vi "Format Coordinates.vi"(11 "1D String Array":string[](array[string])) -> (3 "Coordinates":i32[][](array[numeric]))   [LabVIEW 2019]
doc: "Given a 1D string array of points, turn them into a 2D array of coordinates."
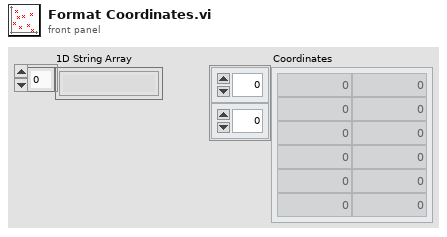
[diagram p1: front panel]
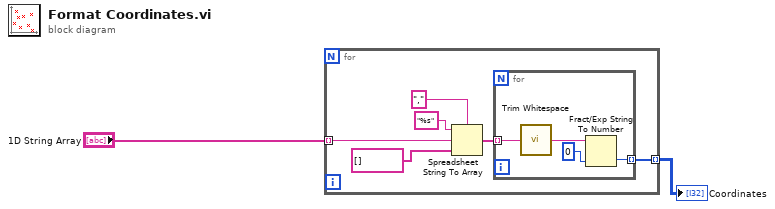
[diagram p0: block diagram]
diagram:
  n1 = for {
    tunnel: "1D String Array" -> [w8] mode=indexing
    tunnel: [w3] -> w2 mode=indexing
    n2 = Spreadsheet String To Array(delimiter (Tab)="," ("delimiter"), format string="%s", spreadsheet string=w8, array type (2D Dbl)=string[] []) -> (array=w5:string[])
    n3 = for {
      tunnel: w5 -> [w12] mode=indexing
      tunnel: [w9] -> w3 mode=indexing
      n4 = call <vilib>:"Trim Whitespace.vi"("string"=w12) -> ("trimmed string"=w11:string)  [unwired: 1 in]
      n5 = Fract/Exp String To Number(string=w11, default (0 dbl)=0 ("default (0 DBL)")) -> (number=w9:i32)  [unwired: 2 in, 1 out]
    }
  }
  "Coordinates" <- w2
